vi "Climb_Pivot_Test.vi"(10 "Joystick_In":T1) -> ()   [LabVIEW 2019]
uses:
  Globals/Climb_Globals.vi
  Subsystems/Climb/Climb_Pivot/Climb_Pivot_Control_States.ctl
  Subsystems/Climb/Climb_Pivot/Climb_Pivot_Cluster.ctl
  Utility_VIs/Joystick_Controls.ctl
panel:
  in  "Pivot_Power":dbl=1.0
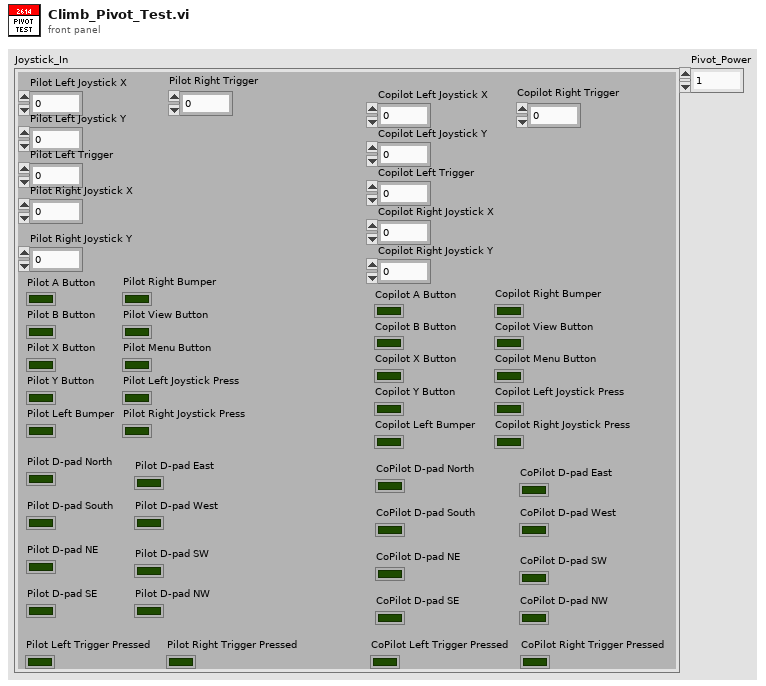
[diagram p1: front panel]
types:
  T1 = typedef "Joystick_Controls.ctl" = cluster{"Pilot Left Joystick X":dbl, "Pilot Left Joystick Y":dbl, "Pilot A Button":bool, "Pilot B Button":bool, "Pilot X Button":bool, "Pilot Y Button":bool, "Pilot Left Bumper":bool, "Pilot Right Bumper":bool, "Pilot View Button":bool, "Pilot Menu Button":bool, "Pilot Left Joystick Press":bool, "Pilot Right Joystick Press":bool, "Pilot Left Trigger":dbl, "Pilot Right Joystick X":dbl, "Pilot Right Joystick Y":dbl, "Pilot Right Trigger":dbl, "Copilot Left Joystick X":dbl, "Copilot Left Joystick Y":dbl, "Copilot A Button":bool, "Copilot B Button":bool, "Copilot X Button":bool, "Copilot Y Button":bool, "Copilot Left Bumper":bool, "Copilot Right Bumper":bool, "Copilot View Button":bool, "Copilot Menu Button":bool, "Copilot Left Joystick Press":bool, "Copilot Right Joystick Press":bool, "Copilot Left Trigger":dbl, "Copilot Right Joystick X":dbl, "Copilot Right Joystick Y":dbl, "Copilot Right Trigger":dbl, "Pilot D-pad North":bool, "Pilot D-pad South":bool, "Pilot D-pad East":bool, "Pilot D-pad West":bool, "Pilot D-pad NE ":bool, "Pilot D-pad SE":bool, "Pilot D-pad SW":bool, "Pilot D-pad NW":bool, "CoPilot D-pad North":bool, "CoPilot D-pad South":bool, "CoPilot D-pad East":bool, "CoPilot D-pad West":bool, "CoPilot D-pad NE":bool, "CoPilot D-pad SE":bool, "CoPilot D-pad SW":bool, "CoPilot D-pad NW":bool, "Pilot Left Trigger Pressed":bool, "Pilot Right Trigger Pressed":bool, "CoPilot Left Trigger Pressed":bool, "CoPilot Right Trigger Pressed":bool}
  T2 = typedef "Climb_Pivot_Cluster.ctl" = cluster{"Up?":bool, "Pivot_Throttle":dbl, "Control_States":T3}
  T3 = typedef "Climb_Pivot_Control_States.ctl" = enum16{"No-Op", "Moving_Down", "Moving_Up", "Manual"}
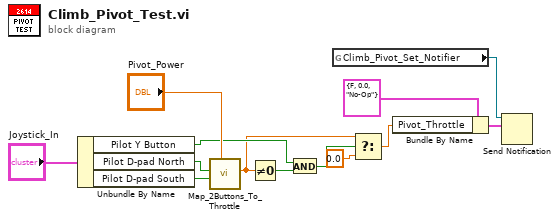
[diagram p0: block diagram]
diagram:
  n1 = Unbundle By Name("Joystick_In") -> ("Pilot Y Button"=w8:bool, "Pilot D-pad North"=w12:bool, "Pilot D-pad South"=w11:bool)
  n2 = call "Map_2Buttons_To_Throttle.vi"("Power"="Pivot_Power", "Down"=w11, "Up"=w12) -> ("Throttle"=w2:dbl)  [unwired: 8 in]
  n3 = Not Equal To 0?(x=w2) -> (x != 0?=w9:bool)
  n4 = And(x=w8, y=w9) -> (x .and. y?=w4:bool)
  n5 = global read "Climb_Globals.vi" "Climb_Pivot_Set_Notifier"() -> (w7:refnum<notifier>)
  n6 = Select(t=w2, s=w4, f=0.0) -> (s? t:f=w3:dbl)
  n7 = Bundle By Name(cluster=T2 {"Up?"=FALSE, "Pivot_Throttle"=0.0, "Control_States"=enum."No-Op"} ("Climb_Pivot_Cluster"), "Pivot_Throttle"=w3) -> (w6:T2)
  n8 = Send Notification(notification=w6, notifier=w7) -> ()  [unwired: 1 in, 2 out]
